vi "Cleanup Session.vi"(8 "error in":errorcluster, 11 "Plugin in":refnum<class "StreamWriter.lvclass">) -> (0 "error out":errorcluster, 3 "Plugin out":refnum<class "StreamWriter.lvclass">)   [LabVIEW 2024, in "StreamWriter.lvlib" / "StreamWriter.lvclass"]
uses:
  StreamWriter.lvclass
  StreamWriter.lvclass/StreamWriter.ctl
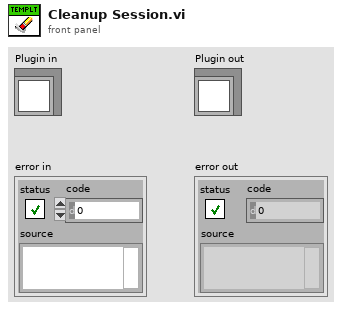
[diagram p1: front panel]
types:
  T1 = typedef "StreamWriter.lvlib/StreamWriter.lvclass/StreamWriter Parameters.ctl" = cluster{"Writer URL":string, "Buffer Size":i32, "Writer Endpoint":refnum<k21>, "Stream Names":string[]}
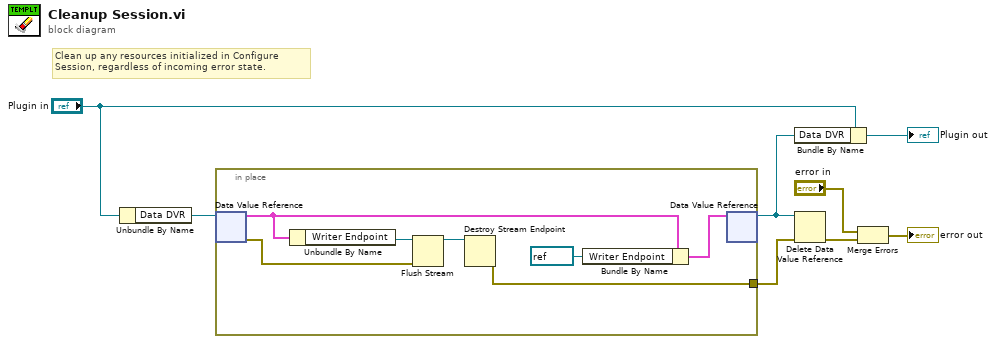
[diagram p0: block diagram]
diagram:
  # "Clean up any resources initialized in Configure Session, regardless of incoming error state."
  n1 = Unbundle By Name("Plugin in") -> ("Data DVR"=w8:refnum<data-value>)
  n2 = in-place {
    in-place-border: [w9] -> w6
    n3 = in-place-dvr #1(w8) -> (w13:T1, w10:errorcluster)
    n4 = Unbundle By Name(w13) -> ("Writer Endpoint"=w14:refnum<k21>)
    n5 = Flush Stream(8:w10, 11:w14) -> (3:w15:refnum<k21>)  [unwired: 2 in, 2 out]
    n6 = Destroy Stream Endpoint(11:w15) -> (0:w9:errorcluster)  [unwired: 1 in]
    n7 = Bundle By Name(cluster=w13, "Writer Endpoint"=refnum<k21> refnum) -> (w11:T1)
    n8 = in-place-dvr #1(w11) -> (w7:refnum<data-value>)  [unwired: 1 out]
  }
  n9 = Bundle By Name(cluster="Plugin in", "Data DVR"=w7) -> (→"Plugin out":refnum<class "StreamWriter.lvclass">)
  n10 = Delete Data Value Reference(data value reference=w7, error in=w6) -> (error out=w5:errorcluster)  [unwired: 1 out]
  n11 = Merge Errors("error in", w5) -> (→"error out":errorcluster)
